vi "Add VI or CTL to lvproj.vi"(8 "error in":errorcluster, 10 "Project Name":string, 11 "Reference of newly created VI or CTL":refnum<vi>) -> (0 "error out":errorcluster)   [LabVIEW 2022 SP3]
doc: "This VI adds the newly created VI or CTL to a project (lvproj).\n\nThis VI assumes that the newly created VI has already been saved to disk (already exists on disk)."
panel:
  # "Development\ncontrols/indicators useful for development and testing, but which are not outputs of the VI"
  # "Input\nInputs to the VI"
  # "Output\nOutputs of the VI"
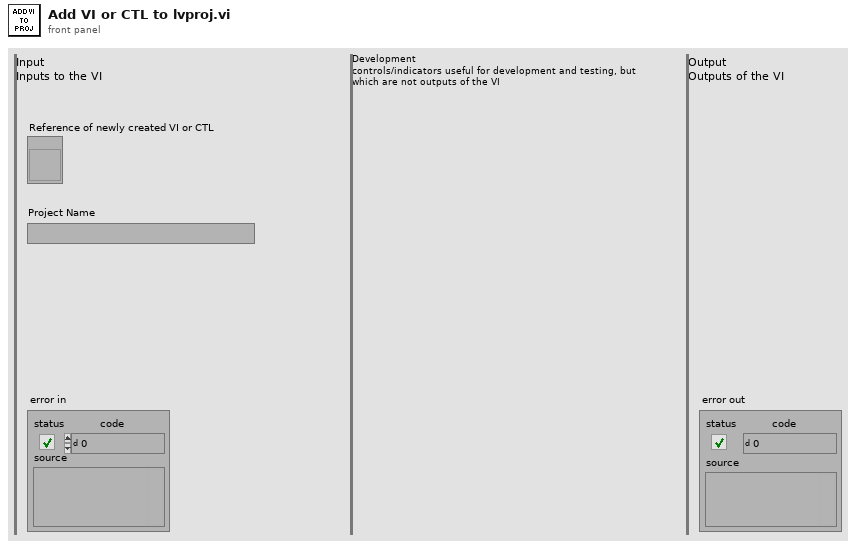
[diagram p1: front panel]
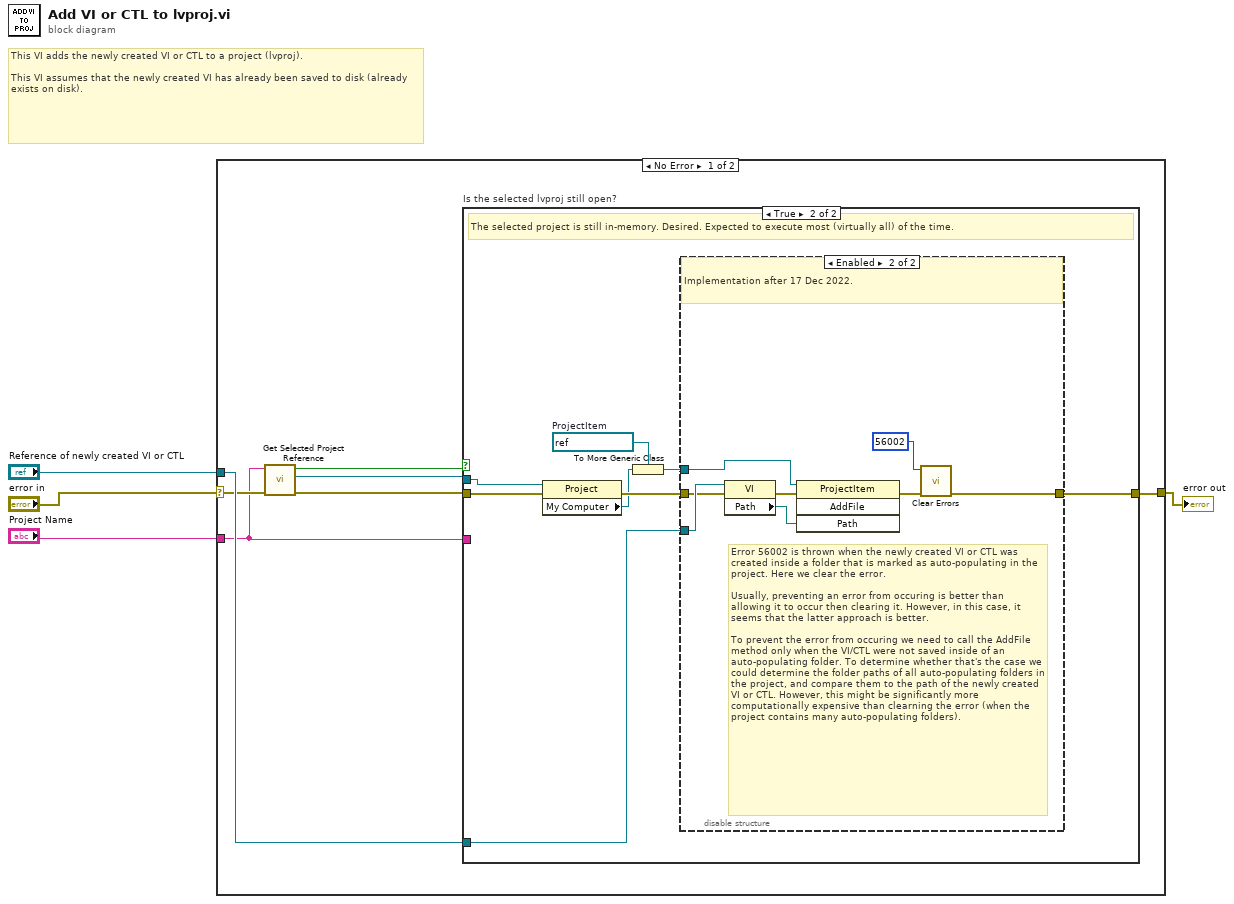
[diagram p0: block diagram]
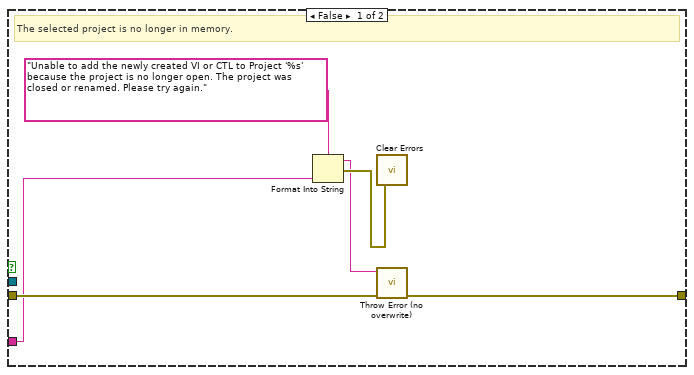
[diagram p2: hidden frame]
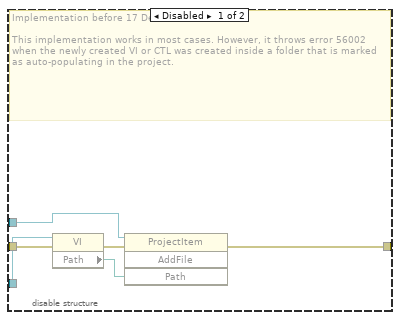
[diagram p3: hidden frame]
diagram:
  # "This VI adds the newly created VI or CTL to a project (lvproj).\n\nThis VI assumes that the newly created VI has already been saved to disk (already exists on disk)."
  n1 = case shown="No Error" "error in" {
    selector: "error in" -> [w9 w40]
    tunnel: [w11 w40] -> w3
    tunnel: "Reference of newly created VI or CTL" -> [w10 _]
    tunnel: "Project Name" -> [w8 _]
    frame No Error {
      n2 = call "Get Selected Project Reference.vi"("error in"=w9, "Selected Project Name"=w8) -> ("error out"=w7:errorcluster, "Project Refnum"=w6:refnum<vi>, "Was Project Found?"=w5:bool)  [unwired: 7 in]
      n3 = case "Is the selected lvproj still open?" shown="True" w5 {
        tunnel: [w16 w23] -> w11
        tunnel: w7 -> [w17 w25]
        tunnel: w6 -> [_ w24]
        tunnel: w10 -> [_ w22]
        tunnel: w8 -> [w13 _]
        frame False {
          # "The selected project is no longer in memory."
          n4 = Format Into String(format string="Unable to add the newly created VI or CTL to Project '%s' because the project is no longer open. The project was closed or renamed. Please try again." ("message"), w13) -> (resulting string=w12:string, error out=w14:errorcluster)  [unwired: 2 in]
          n5 = call <vilib>:"Clear Errors.vi"("error in (no error)"=w14) -> ()  [unwired: 5 in, 2 out]
          n6 = call "Throw Error (no overwrite).vi"("error in"=w17, "Error Message"=w12) -> ("error out"=w16:errorcluster)  [unwired: 9 in]
        }
        frame True {
          w18 = refnum<vi> refnum  # ProjectItem
          # "The selected project is still in-memory. Desired. Expected to execute most (virtually all) of the time."
          n7 = property class="Project"(reference=w24, error in=w25) -> (error out=w20:errorcluster, "My Computer"=w19:refnum<vi>)  [unwired: 1 out]
          n8 = To More Generic Class(target class=w18, reference=w19) -> (generic class reference=w21:refnum<vi>)
          n9 = disable-structure shown="Enabled" {
            disable-tunnel: [w31 w33] -> w23
            disable-tunnel: w22 -> [w30 w38]
            disable-tunnel: w21 -> [w28 w36]
            disable-tunnel: w20 -> [w27 w35]
            frame Disabled {
              # "Implementation before 17 Dec 2022.\n\nThis implementation works in most cases. However, it throws error 56002 when the newly created VI or CTL was created inside a folder that is marked as auto-populating in the project."
              n10 = property class="VI"(reference=w30, error in=w27) -> (error out=w26:errorcluster, "Path"=w29:path)  [unwired: 1 out]
              n11 = invoke class="ProjectItem" method="AddFile"(reference=w28, error in=w26, "Path"=w29) -> (error out=w31:errorcluster)  [unwired: 1 in, 3 out]
            }
            frame Enabled {
              # "Error 56002 is thrown when the newly created VI or CTL was created inside a folder that is marked as auto-populating in the project. Here we clear the error.\n\nUsually, preventing an error from occuring is better than allowing it to occur then clearing it. However, in this case, it seems that the latter approach is better.\n\nTo prevent the error from occuring we need to call the AddFile method only when the VI/CTL were not saved inside of an auto-populating folder. To determine whether that's the case we could determine the folder paths of all auto-populating folders in the project, and compare them to the path of the newly created VI or CTL. However, this might be significantly more computationally expensive than clearning the error (when the project contains many auto-populating folders)."
              # "Implementation after 17 Dec 2022."
              n12 = property class="VI"(reference=w38, error in=w35) -> (error out=w34:errorcluster, "Path"=w37:path)  [unwired: 1 out]
              n13 = invoke class="ProjectItem" method="AddFile"(reference=w36, error in=w34, "Path"=w37) -> (error out=w39:errorcluster)  [unwired: 1 in, 3 out]
              n14 = call <vilib>:"Clear Errors.vi"("error in (no error)"=w39, "specific error code to clear (0: all)"=56002) -> ("error out"=w33:errorcluster)  [unwired: 4 in, 1 out]
            }
          }
        }
      }
    }
    frame Error {
    }
  }
  "error out" <- w3
